vi "Limelight test.vi"() -> ()   [LabVIEW 2019]
doc: "This example shows how to use a digital line to read a limit switch."
panel:
  in  "LED OFF":bool
  in  "LED ON":bool
  in  "stop":bool
  # "Set these inputs before running."
  # "roboRIO Wiring Diagram"
  # "Limit\nSwitch"
  # "COM"
  # "NC"
  # "NO"
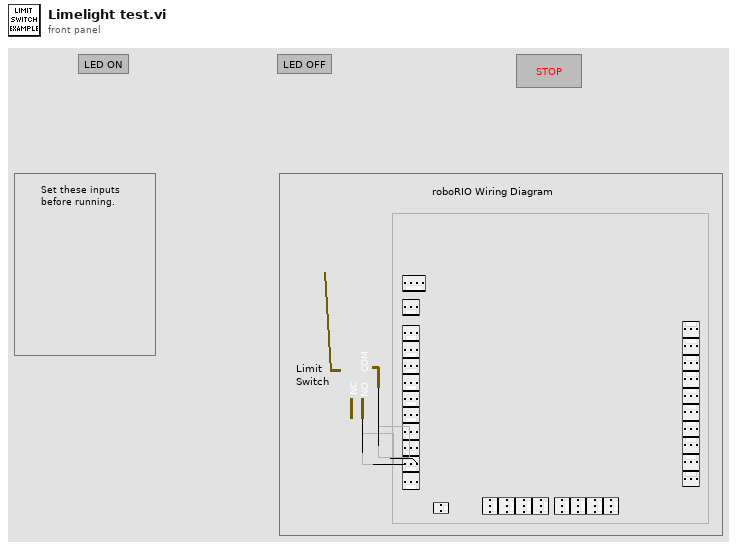
[diagram p1: front panel]
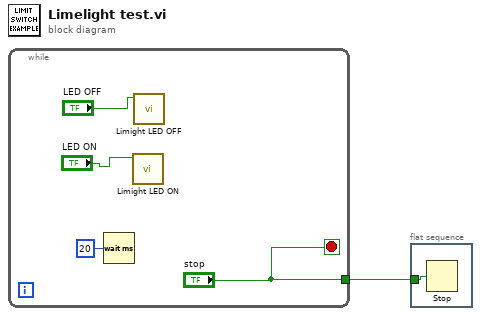
[diagram p0: block diagram]
diagram:
  n1 = while {
    tunnel: ["stop"] -> w1
    stop <- "stop" stop-if-true
    n2 = Wait (ms)(milliseconds to wait=u32 20) -> ()  [unwired: 1 out]
    n3 = call "Limight LED ON.vi"("LED ON"="LED ON") -> ()  [unwired: 11 in]
    n4 = call "Limight LED OFF.vi"("LED OFF"="LED OFF") -> ()  [unwired: 11 in]
  }
  n5 = flat-sequence {
    tunnel: w1 -> [w6]
    frame #0 {
      n6 = Stop(stop? (T)=w6) -> ()
    }
  }
